vi "GetArmCount.vi"(8 "Error In":errorcluster, 11 "Keithley 6482 In":refnum<visa-resource-name>) -> (0 "Error Out":errorcluster, 1 "Infinite?":bool, 2 "Count (1-3000)":u16, 3 "Keithley 6482 Out":refnum<visa-resource-name>)   [LabVIEW 2012, in "Keithley-6482.lvlib"]
uses:
  Keithley-6482.lvlib
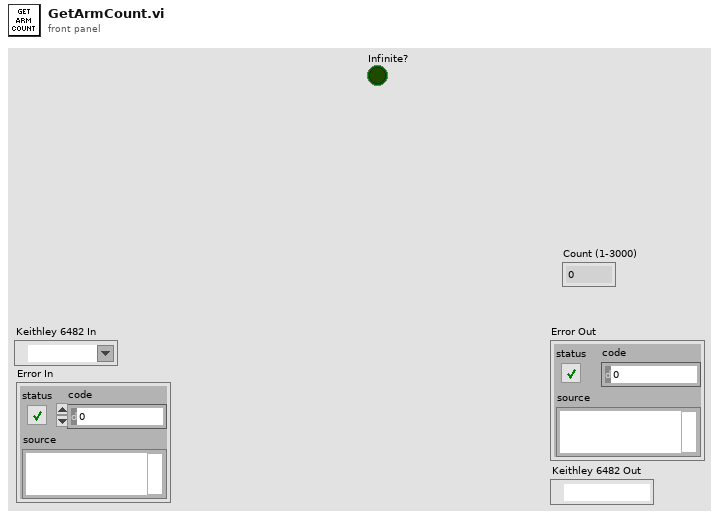
[diagram p1: front panel]
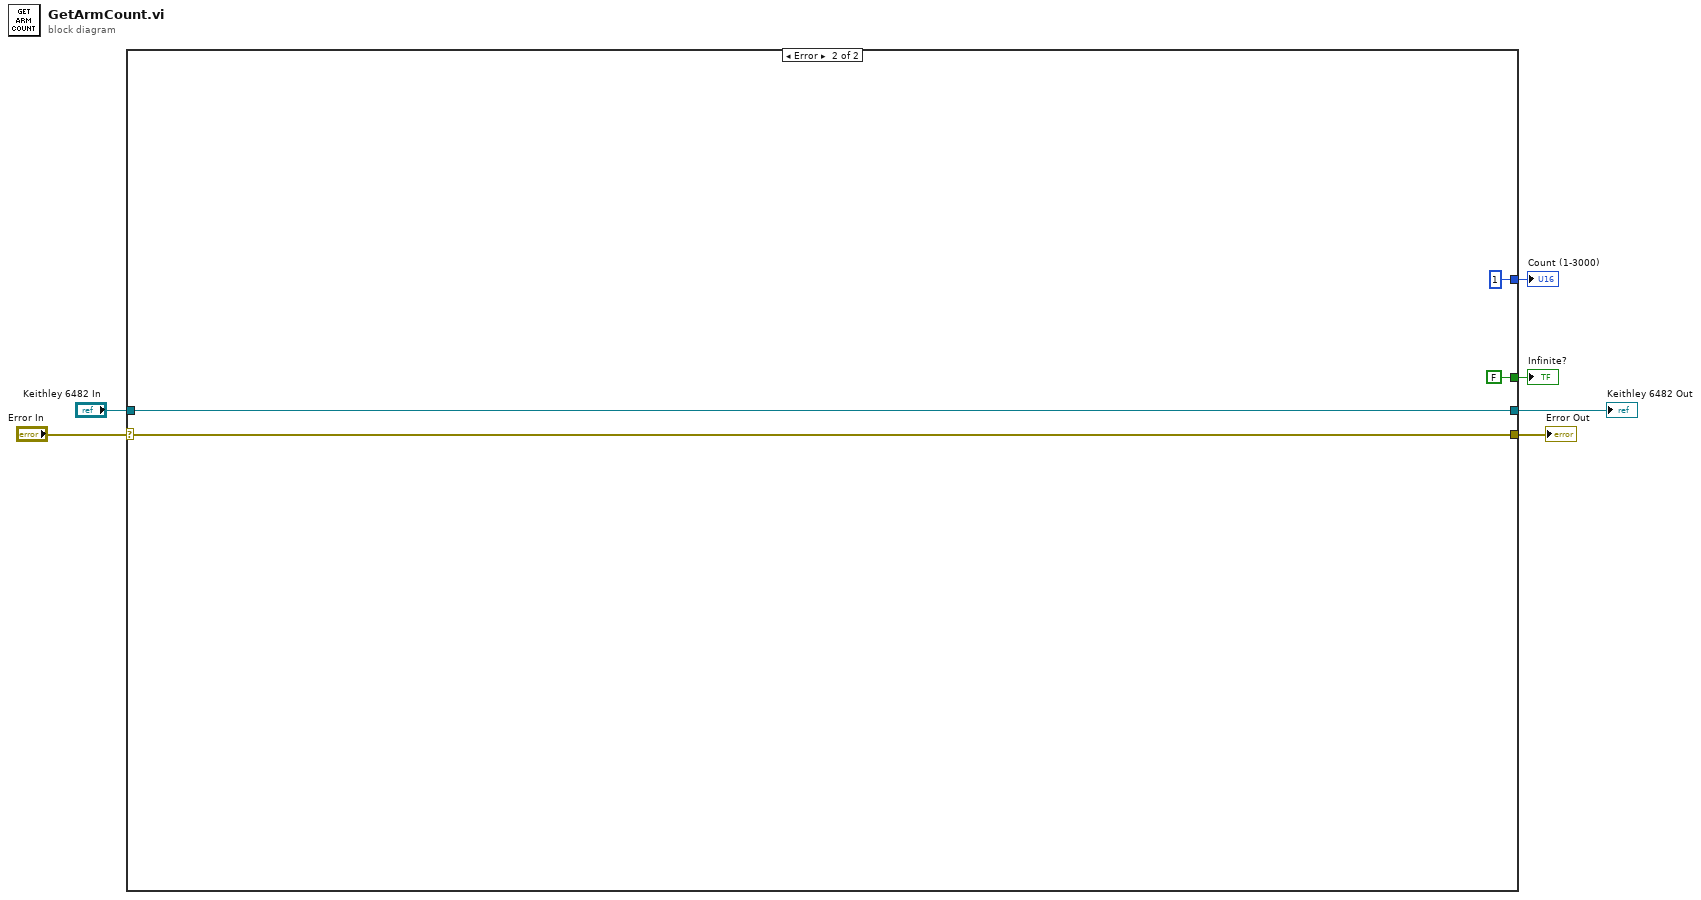
[diagram p0: block diagram]
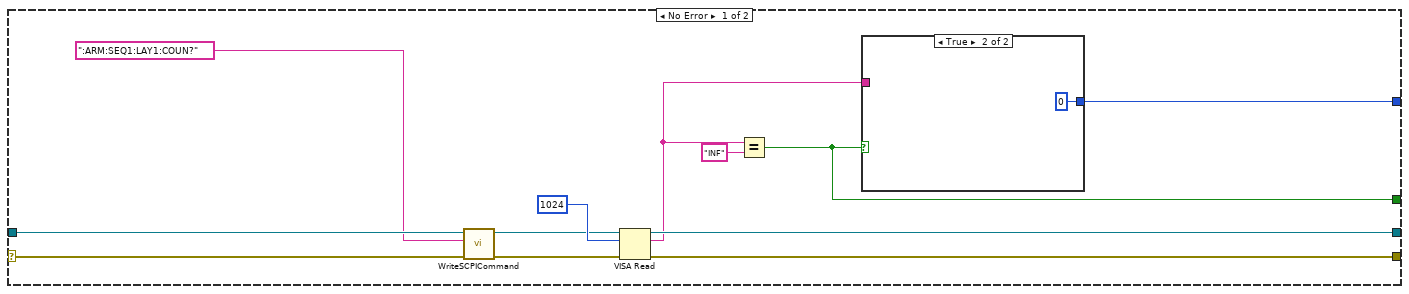
[diagram p2: hidden frame]
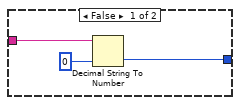
[diagram p3: hidden frame]
diagram:
  n1 = case shown="Error" "Error In" {
    selector: "Error In" -> [w13 w25]
    tunnel: "Keithley 6482 In" -> [w12 w26]
    tunnel: [w18 w25] -> w4
    tunnel: [w17 w26] -> w3
    tunnel: [w11 u16 1] -> w2
    tunnel: [w7 FALSE] -> w1
    frame No Error {
      n2 = call "WriteSCPICommand.vi"("Error In"=w13, "SCPI Command"=":ARM:SEQ1:LAY1:COUN?" ("string"), "Keithley 6482 In"=w12) -> ("Error Out"=w14:errorcluster, "Keithley 6482 Out"=w15:refnum<visa-resource-name>)  [unwired: 7 in]
      n3 = VISA Read(VISA resource name=w15, byte count=u32 1024, error in (no error)=w14) -> (VISA resource name out=w17:refnum<visa-resource-name>, read buffer=w9:string, error out=w18:errorcluster)  [unwired: 1 out]
      n4 = Equal?(x=w9, y="INF") -> (x = y?=w7:bool)
      n5 = case shown="True" w7 {
        tunnel: [w20 u16 0] -> w11
        tunnel: w9 -> [w19 _]
        frame False {
          n6 = Decimal String To Number(string=w19, default (0L)=u16 0) -> (number=w20:u16)  [unwired: 1 in, 1 out]
        }
        frame True {
        }
      }
    }
    frame Error {
    }
  }
  "Error Out" <- w4
  "Keithley 6482 Out" <- w3
  "Count (1-3000)" <- w2
  "Infinite?" <- w1
